vi "SearchFile.vi"() -> ()   [LabVIEW 2022 SP3]
panel:
  out "Filenames":string[](array[string])
  out "Path Array":path[](array[path])
  out "Name":string
  out "Stripped path":path
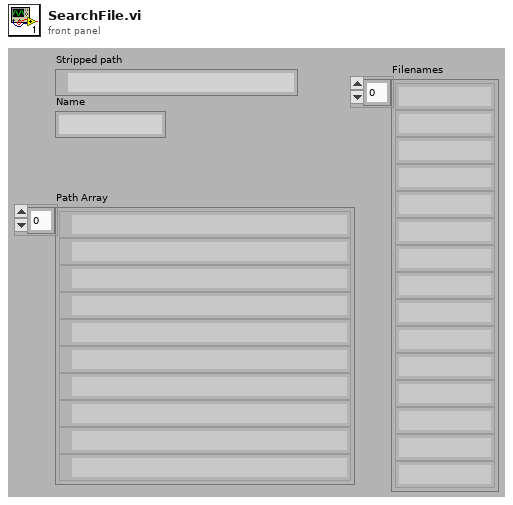
[diagram p1: front panel]
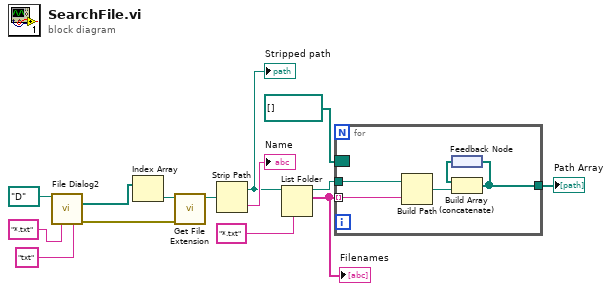
[diagram p0: block diagram]
diagram:
  n1 = call "File Dialog2"("start path"=path "D:/", "pattern (all files)"="*.txt", "pattern label"="txt") -> ("selected paths"=w11:path[], "error out"=w9:errorcluster)  [unwired: 9 in, 2 out]
  n2 = Index Array(array=w11) -> (element=w10:path)  [unwired: 1 in]
  n3 = call <vilib>:"Get File Extension.vi"("error in (no error)"=w9, "file"=w10) -> ("dup file"=w8:path)  [unwired: 5 in, 4 out]
  n4 = Strip Path(path=w8) -> (stripped path=w5:path, name=→"Name":string)
  "Stripped path" <- w5
  n5 = List Folder(path=w5, pattern="*.txt") -> (path out=w3:path, filenames=w2:string[])  [unwired: 2 in, 2 out]
  "Filenames" <- w2
  n6 = for {
    tunnel: w2 -> [w16] mode=indexing
    tunnel: w3 -> [w17]
    border: path[] [] -> [_]
    tunnel: [w15] -> w1
    n7 = Build Path(base path=w17, name or relative path=w16) -> (appended path=w19:path)
    n8 = feedback #1() -> (w18:path[])
    n9 = Build Array (concatenate)(w18, w19) -> (w15:path[])
    n10 = feedback-in #1(w15) -> ()
  }
  "Path Array" <- w1
